vi "Write heartbeat.vi"(10 "IHeartbeat.lvclass":refnum<class "IHeartbeat.lvclass">, 11 "Model in":refnum<class "Model.lvclass">) -> (3 "Model out":refnum<class "Model.lvclass">)   [LabVIEW 2015, in "Model.lvclass"]
uses:
  Model.lvclass
  ComponentTemplateCore/ComponentModel/ComponentModel/Heartbeat/IHeartbeat/IHeartbeat.lvclass
  Model.lvclass/Model.ctl
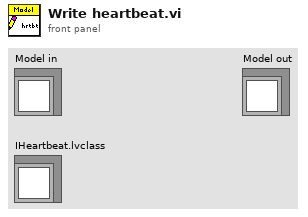
[diagram p1: front panel]
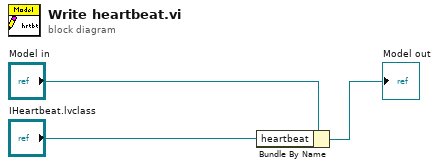
[diagram p0: block diagram]
diagram:
  n1 = Bundle By Name(cluster="Model in", "heartbeat"="IHeartbeat.lvclass") -> (→"Model out":refnum<class "Model.lvclass">)
